vi "zc_db.vi"(0 "action":string, 1 "LabVIEW Web Service Request":refnum<class "Web Request.lvclass"> caption="LabVIEW Web服务请求", 2 "jsren":string, 3 "sp_yijian":string, 4 "key":string, 5 "id":string, 7 "zc_luodi_num":string, 8 "sp_shuoming":string, 11 "didian":string, 13 "shuoming":string, 14 "lc_num":string) -> (15 "error":errorcluster)   [LabVIEW 2017]
uses:
  <vilib>/wsapi/Web Request.lvclass
panel:
  in  "error 4":errorcluster={"status"=TRUE, "code"=254, "source"="您无权申请该流程！"} caption="error"
  in  "error 3":errorcluster={"status"=TRUE, "code"=255, "source"="当前资产不是“入库”状态！"} caption="error"
  out "postdata":string caption="post数据"
  out "error out":errorcluster caption="错误输出"
  # "Web服务请求输入接线端用于调用“Web服务”选板的VI。除非不需要访问该选板，否则不要在连线板上删除这个输入接线端。"
  # "添加至连线板的每一个其他输入控件，在URL中对应于一个输入。如需在接线端模式输出（默认设置）下包含显示控件，则该显示控件必须与连线板相连。"
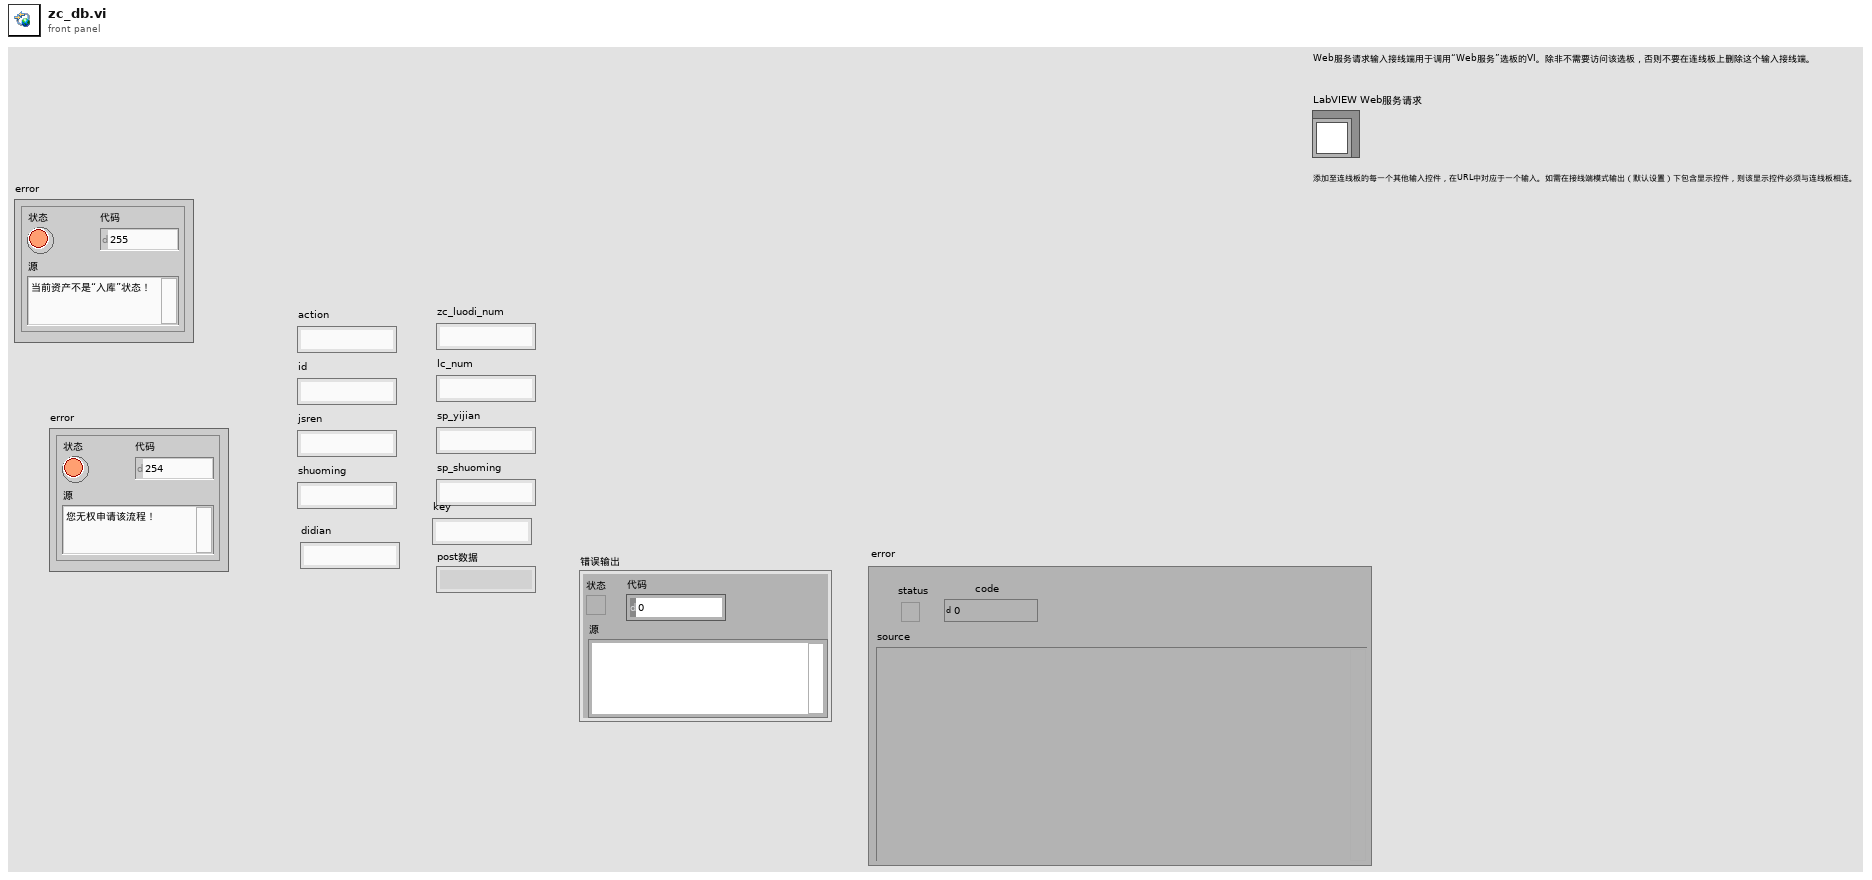
[diagram p1: front panel]
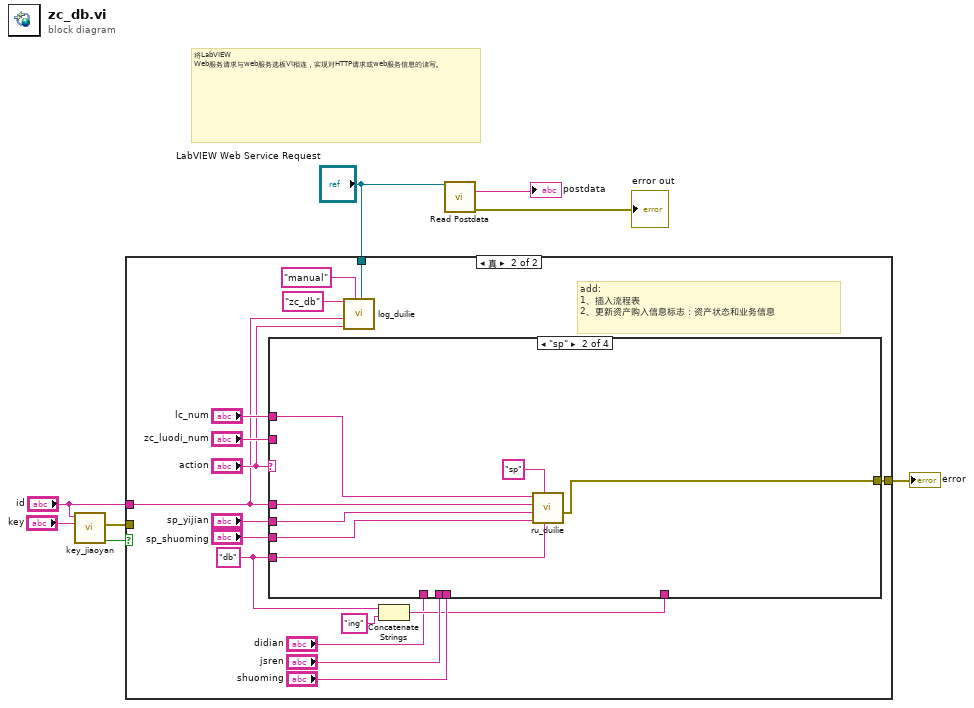
[diagram p0: block diagram]
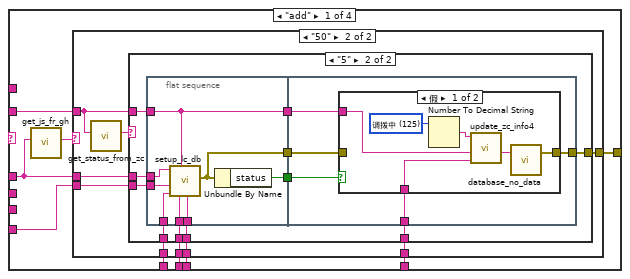
[diagram p3: hidden frame]
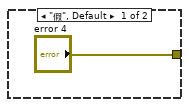
[diagram p4: hidden frame]
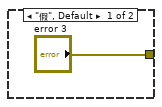
[diagram p5: hidden frame]
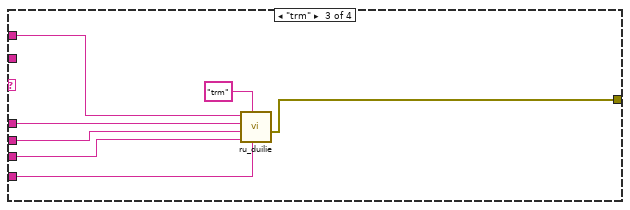
[diagram p7: hidden frame]
diagram:
  # "将LabVIEW Web服务请求与web服务选板VI相连，实现对HTTP请求或web服务信息的读写。"
  n1 = call "key_jiaoyan.vi"("key_client"="key", "gonghao"="id") -> ("jy"=w2:bool, "error"=w1:errorcluster)  [unwired: 8 in]
  n2 = case shown="真" w2 {
    tunnel: [w9 w19] -> w7
    tunnel: "LabVIEW Web Service Request" -> [_ w12]
    tunnel: "id" -> [_ w10]
    tunnel: w1 -> [w9 _]
    frame False {
    }
    frame True {
      w18 = "db" ("yw")
      # "add:\n1、插入流程表\n2、更新资产购入信息标志：资产状态和业务信息"
      n3 = call "log_duilie.vi"("LabVIEW Web Service Request"=w12, "type"="manual", "action"="action", "user"=w10, "yw"="zc_db") -> ()  [unwired: 7 in]
      n4 = Concatenate Strings(w18, "ing" ("字符串")) -> (w16:string)
      n5 = case shown="\"sp\"" "action" {
        tunnel: w10 -> [w27 w82 w89 _]
        tunnel: "zc_luodi_num" -> [w28 _ _ _]
        tunnel: "sp_yijian" -> [_ w80 w87 _]
        tunnel: "sp_shuoming" -> [_ w79 w86 _]
        tunnel: "jsren" -> [w34 _ _ _]
        tunnel: "shuoming" -> [w33 _ _ _]
        tunnel: w18 -> [w32 w78 w85 _]
        tunnel: "lc_num" -> [_ w81 w88 _]
        tunnel: [w31 w77 w84 _] -> w19
        tunnel: w16 -> [w30 _ _ _]
        tunnel: "didian" -> [w29 _ _ _]
        frame "add" {
          n6 = call "get_js_fr_gh.vi"("gonghao"=w27) -> ("juese"=w26:string)  [unwired: 9 in, 1 out]
          n7 = case shown="\"50\"" w26 {
            tunnel: w34 -> [_ w44]
            tunnel: w33 -> [_ w43]
            tunnel: w32 -> [_ w42]
            tunnel: ["error 4" w41] -> w31
            tunnel: w30 -> [_ w40]
            tunnel: w29 -> [_ w39]
            tunnel: w28 -> [_ w38]
            tunnel: w27 -> [_ w36]
            frame "假", Default {
            }
            frame "50" {
              n8 = call "get_status_from_zc.vi"("zc_luodi_num"=w38) -> ("status"=w37:string)  [unwired: 9 in, 1 out]
              n9 = case shown="\"5\"" w37 {
                tunnel: w44 -> [_ w55]
                tunnel: w43 -> [_ w54]
                tunnel: w36 -> [_ w53]
                tunnel: w42 -> [_ w52]
                tunnel: ["error 3" w51] -> w41
                tunnel: w40 -> [_ w50]
                tunnel: w39 -> [_ w49]
                tunnel: w38 -> [_ w48]
                frame "假", Default {
                }
                frame "5" {
                  n10 = flat-sequence {
                    tunnel: w55 -> [w61]
                    tunnel: w54 -> [w60]
                    tunnel: w48 -> [w64]
                    tunnel: w53 -> [w63]
                    tunnel: w52 -> [w62]
                    tunnel: [w64] -> w56
                    tunnel: w49 -> [w59]
                    tunnel: [w58] -> w47
                    tunnel: [w57] -> w46
                    tunnel: w56 -> [w67]
                    tunnel: [w69] -> w51
                    tunnel: w50 -> [w68]
                    tunnel: w47 -> [w66]
                    tunnel: w46 -> [w65]
                    frame #0 {
                      n11 = call "setup_lc_db.vi"("shuoming"=w60, "jsren"=w61, "zc_luodi_num"=w64, "didian"=w59, "yw"=w62, "id"=w63) -> ("error"=w57:errorcluster)  [unwired: 5 in]
                      n12 = Unbundle By Name(w57) -> ("status"=w58:bool)
                    }
                    frame #1 {
                      n13 = case shown="假" w66 {
                        tunnel: [w73 w76] -> w69
                        tunnel: w68 -> [w71 _]
                        tunnel: w67 -> [w70 _]
                        tunnel: w65 -> [_ w76]
                        frame False {
                          w72 = u8 125 items=["待验收"=1, "无需验收"=2, "验收不合格"=3, "待入库"=4, "入库"=5, "领用"=6, "借用"=7, "托管"=8, "接管"=9, "退出"=10, "出库在用"=11, "盘亏"=12, "出售"=13, "报废"=14, "领用中"=120, "退库中"=121, "借用中"=122, "归还中"=123, "转移中"=124, "调拨中"=125, "借调中"=126, "托管中"=127, "终止托管中"=128, "退出中"=129, "处置中"=130] ("状态选择器")
                          n14 = Number To Decimal String(number=w72) -> (decimal integer string=w74:string)  [unwired: 1 in]
                          n15 = call "update_zc_info4.vi"("ywxinxi"=w71, "number"=w70, "status"=w74) -> ("data_str"=w75:string)  [unwired: 8 in]
                          n16 = call "database_no_data.vi"("input"=w75) -> ("error"=w73:errorcluster)  [unwired: 2 in]
                        }
                        frame True {
                        }
                      }
                    }
                  }
                }
              }
            }
          }
        }
        frame "sp" {
          n17 = call "ru_duilie.vi"("yw"=w78, "name"="sp" ("元素"), "sp_shuoming"=w79, "sp_yijian"=w80, "id"=w82, "lc_num"=w81) -> ("error"=w77:errorcluster)  [unwired: 5 in]
        }
        frame "trm" {
          n18 = call "ru_duilie.vi"("yw"=w85, "name"="trm" ("元素"), "sp_shuoming"=w86, "sp_yijian"=w87, "id"=w89, "lc_num"=w88) -> ("error"=w84:errorcluster)  [unwired: 5 in]
        }
        frame Default {
        }
      }
    }
  }
  "error" <- w7
  n19 = call <vilib>:"Read Postdata.vi"("LabVIEW Web Service Request"="LabVIEW Web Service Request") -> ("postdata"=→"postdata":string, "error out"=→"error out":errorcluster)  [unwired: 12 in, 1 out]
